vi "XCP Initialize DAQ List 2.vi"(0 "Measurement List":string[](array[string]), 1 "DTO IDs":u32[](array[numeric]), 2 "Save Database":bool, 5 "ECU ref in":T2, 7 "CAN Interface":refnum<k21>, 9 "Sample Rate (10 Hz)":dbl=10.0, 11 "error in (no error)":errorcluster, 12 "Special Flag":T1) -> (4 "DAQList out":refnum<class "DAQList.lvclass">, 15 "error out":errorcluster)   [LabVIEW 2019, in "XCP_DaqDtoId.lvlib" / "DAQList.lvclass"]
uses:
  DAQList.lvclass
  <vilib>/ECUMC/ECUMC.llb/MC Reference.ctt
  TypeDef/SpecialFlag.ctl
  DAQList.lvclass/DAQList.ctl
  <vilib>/ECUMC/ECUMC.lvlib
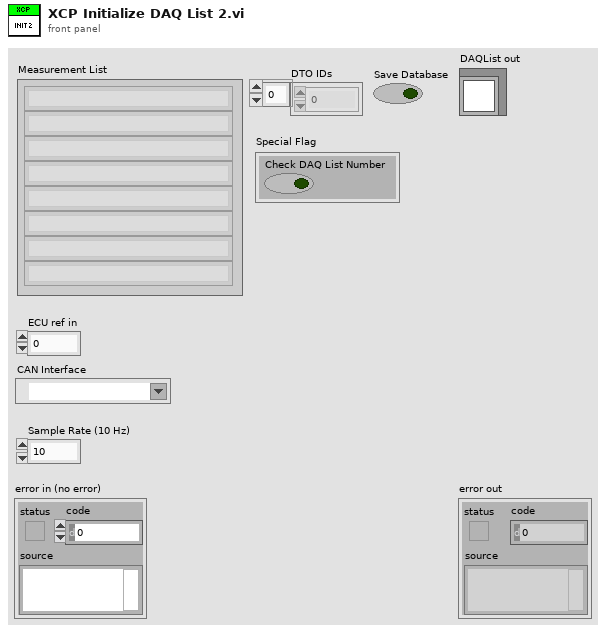
[diagram p1: front panel]
types:
  T1 = typedef "XCP_DaqDtoId.lvlib/DAQList.lvclass/SpecialFlag.ctl" = cluster{"Check DAQ List Number":bool}
  T2 = typedef "ECUMC.lvlib/MC Reference.ctt" = u32
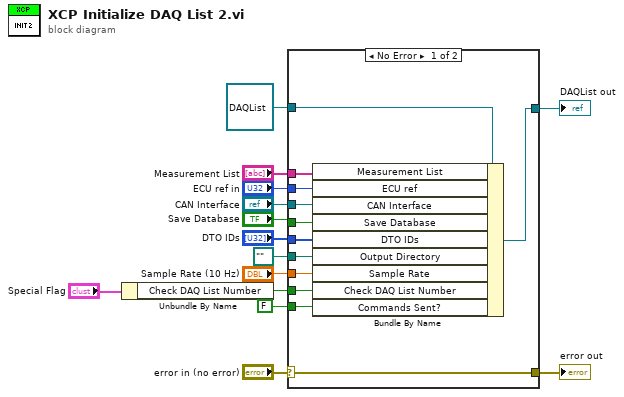
[diagram p0: block diagram]
diagram:
  n1 = Unbundle By Name("Special Flag") -> ("Check DAQ List Number"=w2:bool)
  n2 = case shown="No Error" "error in (no error)" {
    selector: "error in (no error)" -> [w22 w28]
    tunnel: [w22 w28] -> w13
    tunnel: [w16 w27] -> w12
    tunnel: refnum<class "DAQList.lvclass"> refnum ("DAQList out") -> [w26 w27]
    tunnel: "Measurement List" -> [w25 _]
    tunnel: "ECU ref in" -> [w24 _]
    tunnel: "CAN Interface" -> [w23 _]
    tunnel: "Save Database" -> [w21 _]
    tunnel: path "" ("Database Base Path") -> [w20 _]
    tunnel: "DTO IDs" -> [w19 _]
    tunnel: "Sample Rate (10 Hz)" -> [w18 _]
    tunnel: w2 -> [w17 _]
    tunnel: FALSE ("Commands Sent?") -> [w15 _]
    frame No Error {
      n3 = Bundle By Name(cluster=w26, "Measurement List"=w25, "ECU ref"=w24, "CAN Interface"=w23, "Save Database"=w21, "DTO IDs"=w19, "Output Directory"=w20, "Sample Rate"=w18, "Check DAQ List Number"=w17, "Commands Sent?"=w15) -> (w16:refnum<class "DAQList.lvclass">)
    }
    frame Error {
    }
  }
  "error out" <- w13
  "DAQList out" <- w12
